vi "LEBITVacuum.ParseDBArray.vi"(1 "DBArray":string[][](array[string])) -> (9 "Special":string[](array[string]), 10 "nickname":string[](array[string]), 11 "CondSpecial2DArray":string[][](array[string]), 12 "monValuePLC":string[](array[string]), 13 "SpecialIndex":i32[](array[numeric]), 14 "setValuePLC":string[](array[string]), 15 "SetValue":i16[](array[numeric]), 16 "setValuePLCServiceID":i32[](array[numeric]), 17 "SetValueServiceID":i32[](array[numeric]), 18 "MonValueServiceID":i32[](array[numeric]), 19 "enableValuePLC":string[](array[string]))   [LabVIEW 2014, in "LEBITVacuum.lvlib"]
uses:
  LEBITVacuum.lvlib
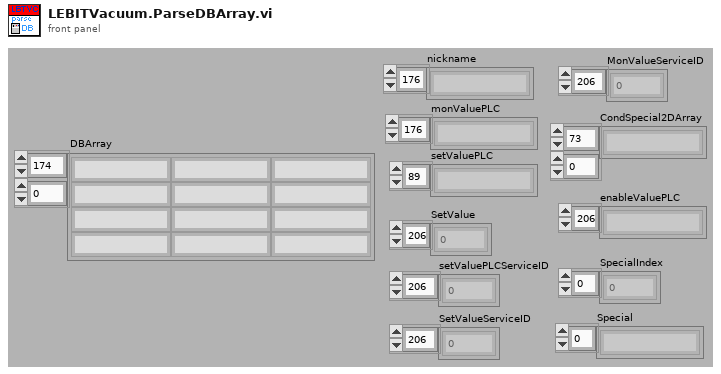
[diagram p1: front panel]
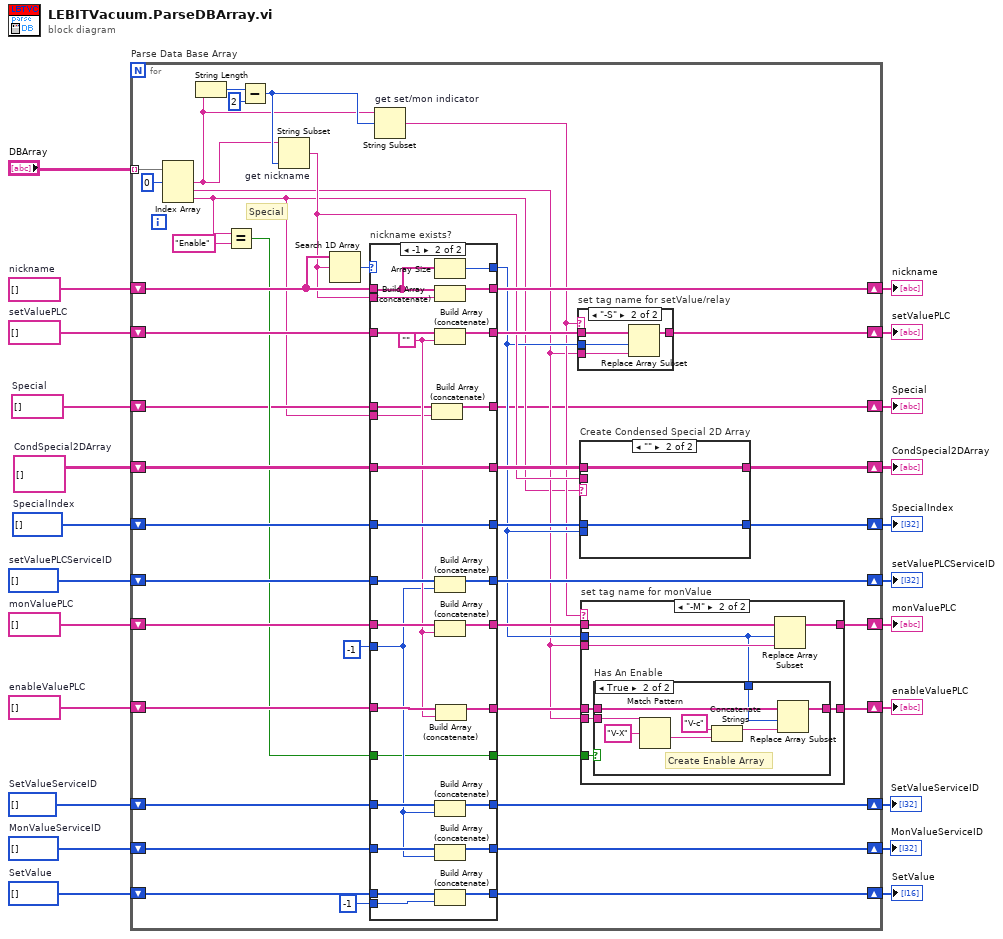
[diagram p0: block diagram]
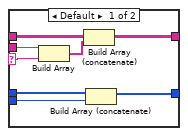
[diagram p2: hidden frame]
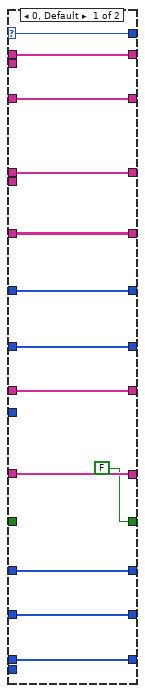
[diagram p5: hidden frame]
diagram:
  w2 = string[] []  # Special
  w4 = string[] []  # enableValuePLC
  w8 = i32[] []  # SpecialIndex
  w9 = string[][] []  # CondSpecial2DArray
  w10 = i16[] []  # SetValue
  w19 = i32[] []  # MonValueServiceID
  w20 = i32[] []  # SetValueServiceID
  w21 = string[] []  # monValuePLC
  w18 = i32[] []  # setValuePLCServiceID
  w22 = string[] []  # setValuePLC
  w23 = string[] []  # nickname
  n1 = for "Parse Data Base Array" {
    tunnel: "DBArray" -> [w67] mode=indexing
    shift-right: [w54] -> w17
    shift-left: w23 -> [w61]
    shift-right: [w53] -> w16
    shift-left: w22 -> [w60]
    shift-right: [w51] -> w15
    shift-left: w18 -> [w52]
    shift-right: [w49] -> w14
    shift-left: w21 -> [w59]
    shift-right: [w48] -> w13
    shift-left: w20 -> [w58]
    shift-right: [w47] -> w12
    shift-left: w19 -> [w57]
    shift-right: [w45] -> w5
    shift-left: w10 -> [w46]
    shift-right: [w42] -> w7
    shift-left: w9 -> [w44]
    shift-right: [w38] -> w6
    shift-left: w8 -> [w40]
    shift-right: [w33] -> w3
    shift-left: w4 -> [w35]
    shift-right: [w24] -> w1
    shift-left: w2 -> [w26]
    # "Special"
    n2 = Index Array(array=w67, index #1=0 ("index")) -> (element #1=w30:string, element #2=w32:string, element #3=w25:string)  [unwired: 2 in]
    n3 = String Length(string=w30) -> (length=w65:i32)
    n4 = Equal?(x=w25, y="Enable") -> (x = y?=w27:bool)
    n5 = Subtract(x=w65, y=2) -> (x-y=w63:i32)
    n6 = String Subset "get nickname"(string=w30, length (rest)=w63) -> (substring=w41:string)  [unwired: 1 in]
    n7 = Search 1D Array(1D array=w61, element=w41) -> (index of element=w62:i32)  [unwired: 1 in]
    n8 = case "nickname exists?" shown="-1" w62 {
      selector: w62 -> [w103 _]
      tunnel: w61 -> [w109 w125]
      tunnel: w41 -> [_ w136]
      tunnel: [w109 w135] -> w54
      tunnel: w60 -> [w108 w134]
      tunnel: w52 -> [w107 w133]
      tunnel: w59 -> [w106 w132]
      tunnel: w58 -> [w105 w131]
      tunnel: w57 -> [w104 w130]
      tunnel: [w108 w129] -> w55
      tunnel: [w107 w126] -> w51
      tunnel: [w106 w127] -> w50
      tunnel: [w105 w128] -> w48
      tunnel: [w104 w122] -> w47
      tunnel: -1 -> [_ w115]
      tunnel: [w103 w124] -> w37
      tunnel: w46 -> [w102 w123]
      tunnel: [w102 w121] -> w45
      tunnel: w44 -> [w101 w120]
      tunnel: [w101 w120] -> w43
      tunnel: w40 -> [w100 w119]
      tunnel: [w100 w119] -> w39
      tunnel: w35 -> [w99 w118]
      tunnel: [w99 w116] -> w34
      tunnel: i16 -1 -> [_ w114]
      tunnel: [FALSE w113] -> w29
      tunnel: w27 -> [_ w113]
      tunnel: w26 -> [w97 w112]
      tunnel: w25 -> [_ w111]
      tunnel: [w97 w110] -> w24
      frame 0, Default {
      }
      frame -1 {
        w117 = ""
        n9 = Build Array (concatenate)(w112, w111) -> (w110:string[])
        n10 = Array Size(array=w125) -> (size(s)=w124:i32)
        n11 = Build Array (concatenate)(w125, w136) -> (w135:string[])
        n12 = Build Array (concatenate)(w134, w117) -> (w129:string[])
        n13 = Build Array (concatenate)(w133, w115) -> (w126:i32[])
        n14 = Build Array (concatenate)(w132, w117) -> (w127:string[])
        n15 = Build Array (concatenate)(w131, w115) -> (w128:i32[])
        n16 = Build Array (concatenate)(w130, w115) -> (w122:i32[])
        n17 = Build Array (concatenate)(w123, w114) -> (w121:i16[])
        n18 = Build Array (concatenate)(w118, w117) -> (w116:string[])
      }
    }
    n19 = String Subset "get set/mon indicator"(string=w30, offset (0)=w63) -> (substring=w36:string)  [unwired: 1 in]
    n20 = case "set tag name for setValue/relay" shown="\"-S\"" w36 {
      tunnel: w55 -> [w137 w141]
      tunnel: w37 -> [_ w138]
      tunnel: w32 -> [_ w140]
      tunnel: [w137 w139] -> w53
      frame Default {
      }
      frame "-S" {
        n21 = Replace Array Subset(array=w141, new element=w140, index=w138) -> (w139:string[])
      }
    }
    n22 = case "Create Condensed Special 2D Array" shown="\"\"" w25 {
      selector: w25 -> [w71 _]
      tunnel: w43 -> [w75 w77]
      tunnel: [w74 w77] -> w42
      tunnel: w41 -> [w72 _]
      tunnel: w39 -> [w70 w76]
      tunnel: [w69 w76] -> w38
      tunnel: w37 -> [w68 _]
      frame Default {
        n23 = Build Array(w72, w71) -> (w73:string[])
        n24 = Build Array (concatenate)(w75, w73) -> (w74:string[][])
        n25 = Build Array (concatenate)(w70, w68) -> (w69:i32[])
      }
      frame "" {
      }
    }
    n26 = case "set tag name for monValue" shown="\"-M\"" w36 {
      tunnel: w50 -> [w79 w87]
      tunnel: w37 -> [_ w82]
      tunnel: w32 -> [_ w86]
      tunnel: [w79 w85] -> w49
      tunnel: w34 -> [w78 w84]
      tunnel: [w78 w83] -> w33
      tunnel: w32 -> [_ w81]
      tunnel: w29 -> [_ w80]
      frame Default {
      }
      frame "-M" {
        n27 = case "Has An Enable" shown="True" w80 {
          tunnel: w84 -> [w88 w96]
          tunnel: [w88 w95] -> w83
          tunnel: w82 -> [_ w94]
          tunnel: w81 -> [_ w93]
          frame False {
          }
          frame True {
            # "Create Enable Array"
            n28 = Match Pattern(string=w93, regular expression="V-X") -> (after substring=w89:string)  [unwired: 1 in, 3 out]
            n29 = Concatenate Strings("V-c" ("regular expression"), w89) -> (w91:string)
            n30 = Replace Array Subset(array=w96, new element=w91, index=w94) -> (w95:string[])
          }
        }
        n31 = Replace Array Subset(array=w87, new element=w86, index=w82) -> (w85:string[])
      }
    }
  }
  "nickname" <- w17
  "setValuePLC" <- w16
  "setValuePLCServiceID" <- w15
  "monValuePLC" <- w14
  "SetValueServiceID" <- w13
  "MonValueServiceID" <- w12
  "CondSpecial2DArray" <- w7
  "SpecialIndex" <- w6
  "SetValue" <- w5
  "enableValuePLC" <- w3
  "Special" <- w1
